vi "ReplaceName.vi"(8 "error in (no error)":errorcluster, 10 "response":T1, 11 "BaseResponder in":refnum<class "BaseResponder.lvclass">) -> (0 "error out":errorcluster, 2 "response out":T1, 3 "BaseResponder out":refnum<class "BaseResponder.lvclass">)   [LabVIEW 2013, in "BaseResponder.lvclass"]
doc: "Replaces the \"Sender\" field of the response with the name of the responder"
uses:
  BaseResponder.lvclass
  response.ctl
  driver_status.ctl
  BaseResponder.lvclass/BaseResponder.ctl
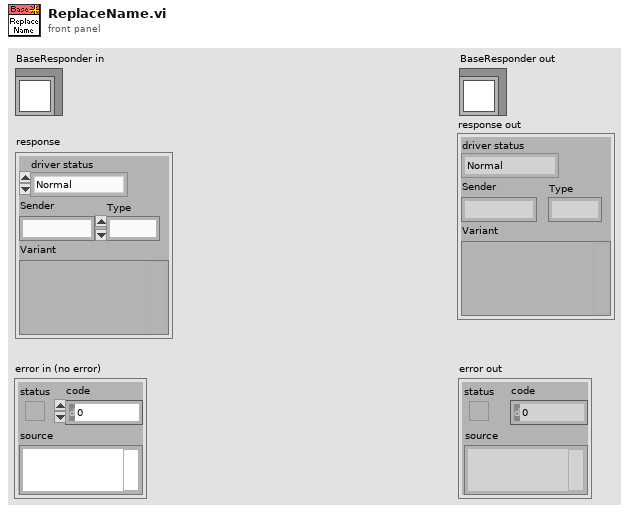
[diagram p1: front panel]
types:
  T1 = typedef "response.ctl" = cluster{"driver status":T2, "Sender":string, "Type":i32, "Variant":variant}
  T2 = typedef "driver_status.ctl" = enum16{"Normal", "Startup", "Connection lost", "Reconnected", "Timeout", "Idle", "Busy"}
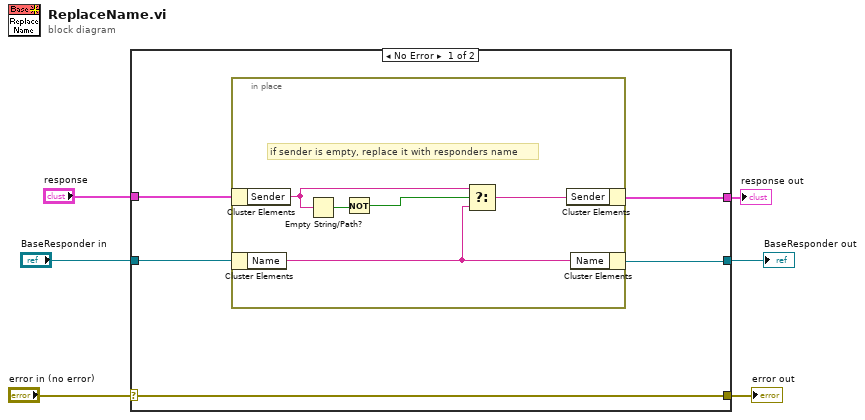
[diagram p0: block diagram]
diagram:
  n1 = case shown="No Error" "error in (no error)" {
    selector: "error in (no error)" -> [w11 w19]
    tunnel: [w11 w19] -> w5
    tunnel: [w8 w18] -> w3
    tunnel: "BaseResponder in" -> [w10 w18]
    tunnel: "response" -> [w9 w17]
    tunnel: [w7 w17] -> w1
    frame No Error {
      n2 = in-place "In Place Element Structure" {
        # "if sender is empty, replace it with responders name"
        n3 = in-place-cluster #1(w9) -> ("Sender"=w16:string)
        n4 = in-place-cluster #2(w10) -> ("Name"=w13:string)
        n5 = Empty String/Path?(string/path=w16) -> (empty?=w15:bool)
        n6 = Not(x=w15) -> (.not. x?=w14:bool)
        n7 = Select(t=w16, s=w14, f=w13) -> (s? t:f=w12:string)
        n8 = in-place-cluster #1("Sender"=w12) -> (w7:T1)
        n9 = in-place-cluster #2("Name"=w13) -> (w8:refnum<class "BaseResponder.lvclass">)
      }
    }
    frame Error {
    }
  }
  "error out" <- w5
  "BaseResponder out" <- w3
  "response out" <- w1
